vi "CreateInputsNode.vi"(8 "Error In":errorcluster, 10 "Pattern":T1, 11 "DOM Document":refnum<k20>) -> (0 "Error out":errorcluster, 3 "Inputs Node":refnum<k20>)   [LabVIEW 2012, in "Virtual-PGA.lvlib"]
uses:
  Virtual-PGA.lvlib
  Public/Controls/Pattern.ctl
  Public/Controls/Input.ctl
  <resource>/objmgr/DOMUserDefRef.rc
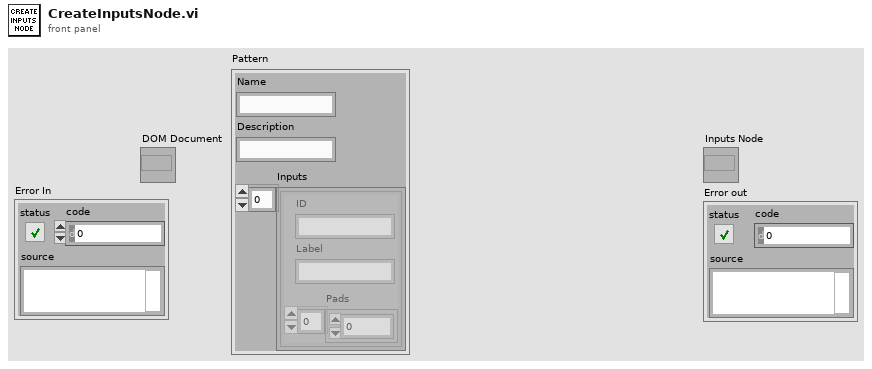
[diagram p1: front panel]
types:
  T1 = typedef "Virtual-PGA.lvlib/Pattern.ctl" = cluster{"Name":string, "Description":string, "Inputs":T2[]}
  T2 = typedef "Virtual-PGA.lvlib/Input.ctl" = cluster{"ID":string, "Label":string, "Pads":u32[]}
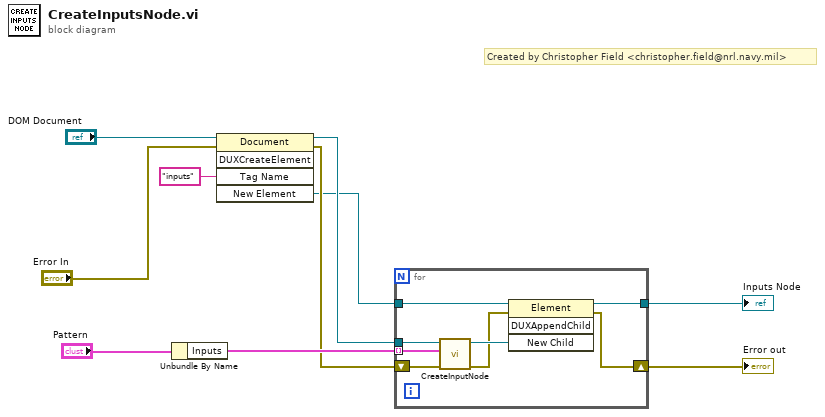
[diagram p0: block diagram]
diagram:
  # "Created by Christopher Field <christopher.field@nrl.navy.mil>"
  n1 = Unbundle By Name("Pattern") -> ("Inputs"=w4:T2[])
  n2 = invoke class="Document" method="DUXCreateElement"(reference="DOM Document", error in="Error In", "Tag Name"="inputs") -> (reference out=w3:refnum<k20>, error out=w2:errorcluster, "New Element"=w1:refnum<k20>)  [unwired: 2 in, 2 out]
  n3 = for {
    tunnel: w4 -> [w16] mode=indexing
    tunnel: w3 -> [w15]
    tunnel: w1 -> [w13]
    tunnel: [w12] -> w8
    shift-right: [w11] -> w7
    shift-left: w2 -> [w14]
    n4 = call "CreateInputNode.vi"("Error In"=w14, "Input"=w16, "DOM Document"=w15) -> ("Error Out"=w17:errorcluster, "Input Node"=w18:refnum<k20>)  [unwired: 7 in]
    n5 = invoke class="Element" method="DUXAppendChild"(reference=w13, error in=w17, "New Child"=w18) -> (reference out=w12:refnum<k20>, error out=w11:errorcluster)  [unwired: 1 in, 2 out]
  }
  "Inputs Node" <- w8
  "Error out" <- w7
